vi "Main.vi"() -> ()   [LabVIEW 2022 SP3]
doc: "This template is for the Queued Message Handler design pattern.\n\nThe Event Handling Loop generates messages based on user interface actions.\n\nThe Message Handling Loop processes messages generated by the Event Handling Loop, or by other messages. The messages are string values, so new messages can be added easily to the Message Cases case structure in the Message Handling Loop. Each message cluster can also provide an optional value for Message Data, which is a variant that can be converted to whatever message-specific data is required."
uses:
  controls/UI Data.ctl
  support/Message Queue/Enqueue Message (Single).vi
  <vilib>/Utility/error.llb/Error Cluster From Error Code.vi
  <vilib>/ErrorRing/Error Ring.xnode
  support/Message Queue/Message Queue.lvlib
  support/User Event - Stop/User Event - Stop.lvlib
  support/User Event - ConnectionEvent/User Event - ConnectionEvent.lvlib
panel:
  out "sensors":dbl[](array[numeric])
  in  "Clear Console":bool
  in  "Restart Remote":bool
  in  "Network DAQ Rate (ms)":u32=500
  in  "Ignition Safety":bool
  in  "Ignition":bool
  in  "Deactuate 5":bool
  in  "Deactuate 4":bool
  in  "Deactuate 3":bool
  in  "Deactuate 2":bool
  in  "Deactuate 1":bool
  in  "Actuate 5":bool
  in  "Actuate 4":bool
  in  "Actuate 3":bool
  in  "Actuate 2":bool
  out "Ignition State":bool
  out "Switch 5":bool
  out "Switch 4":bool
  out "Switch 3":bool
  out "Switch 2":bool
  out "Switch 1":bool
  out "Pressure Transducers":waveform(dbl)[](graph)
  out "Temperature":waveform(dbl)[](graph)
  out "Load Cells & Strain Gauges":waveform(dbl)[](graph)
  out "Console":string
  in  "Disconnect":bool
  in  "Port":dbl=25005.0
  in  "IP Address":string="192.168.1.114"
  in  "Actuate 1":bool
  in  "Connect":bool
  in  "Exit":bool
  # "LC 0"
  # "LC 1"
  # "LC 2"
  # "LC 3"
  # "SG 0"
  # "SG 1"
  # "TC 0"
  # "TC 1"
  # "TC 2"
  # "TC 3"
  # "PT 0"
  # "PT 1"
  # "PT 2"
  # "PT 3"
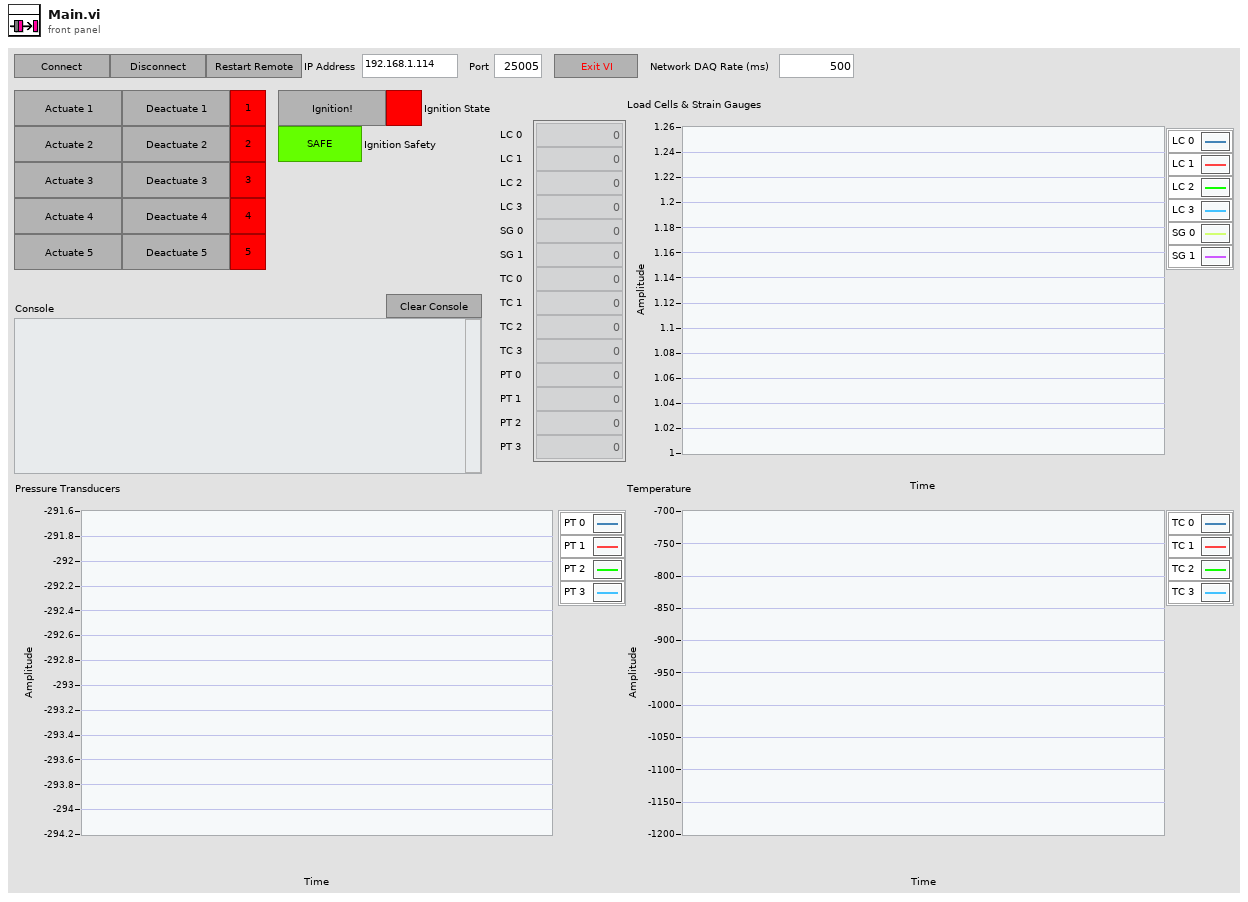
[diagram p1: front panel]
types:
  T1 = cluster{"ConnectionStatus":enum16{"Nothing", "Disconnect", "Connect", "Error"}}
  T2 = typedef "UI Data.ctl" = cluster{"Connect Ref":refnum<vi>, "Disconnect Ref":refnum<vi>, "Console Ref":refnum<vi>, "Exit Button Ref":refnum<vi>, "TCP Network Connection Refnum":refnum<k5>}
  T3 = typedef "Message Queue.lvlib/All Message Queues.ctl" = cluster{"UI":refnum<queue>}
  T4 = cluster{"command":string, "driver":i32, "value":i32}
  T5 = cluster{"[0]":bool, "[1]":bool, "[2]":bool, "[3]":bool, "[4]":bool, "[5]":bool, "[6]":bool, "[7]":bool, "[8]":bool}
  T6 = enum16{"Nothing", "Disconnect", "Connect", "Error"}
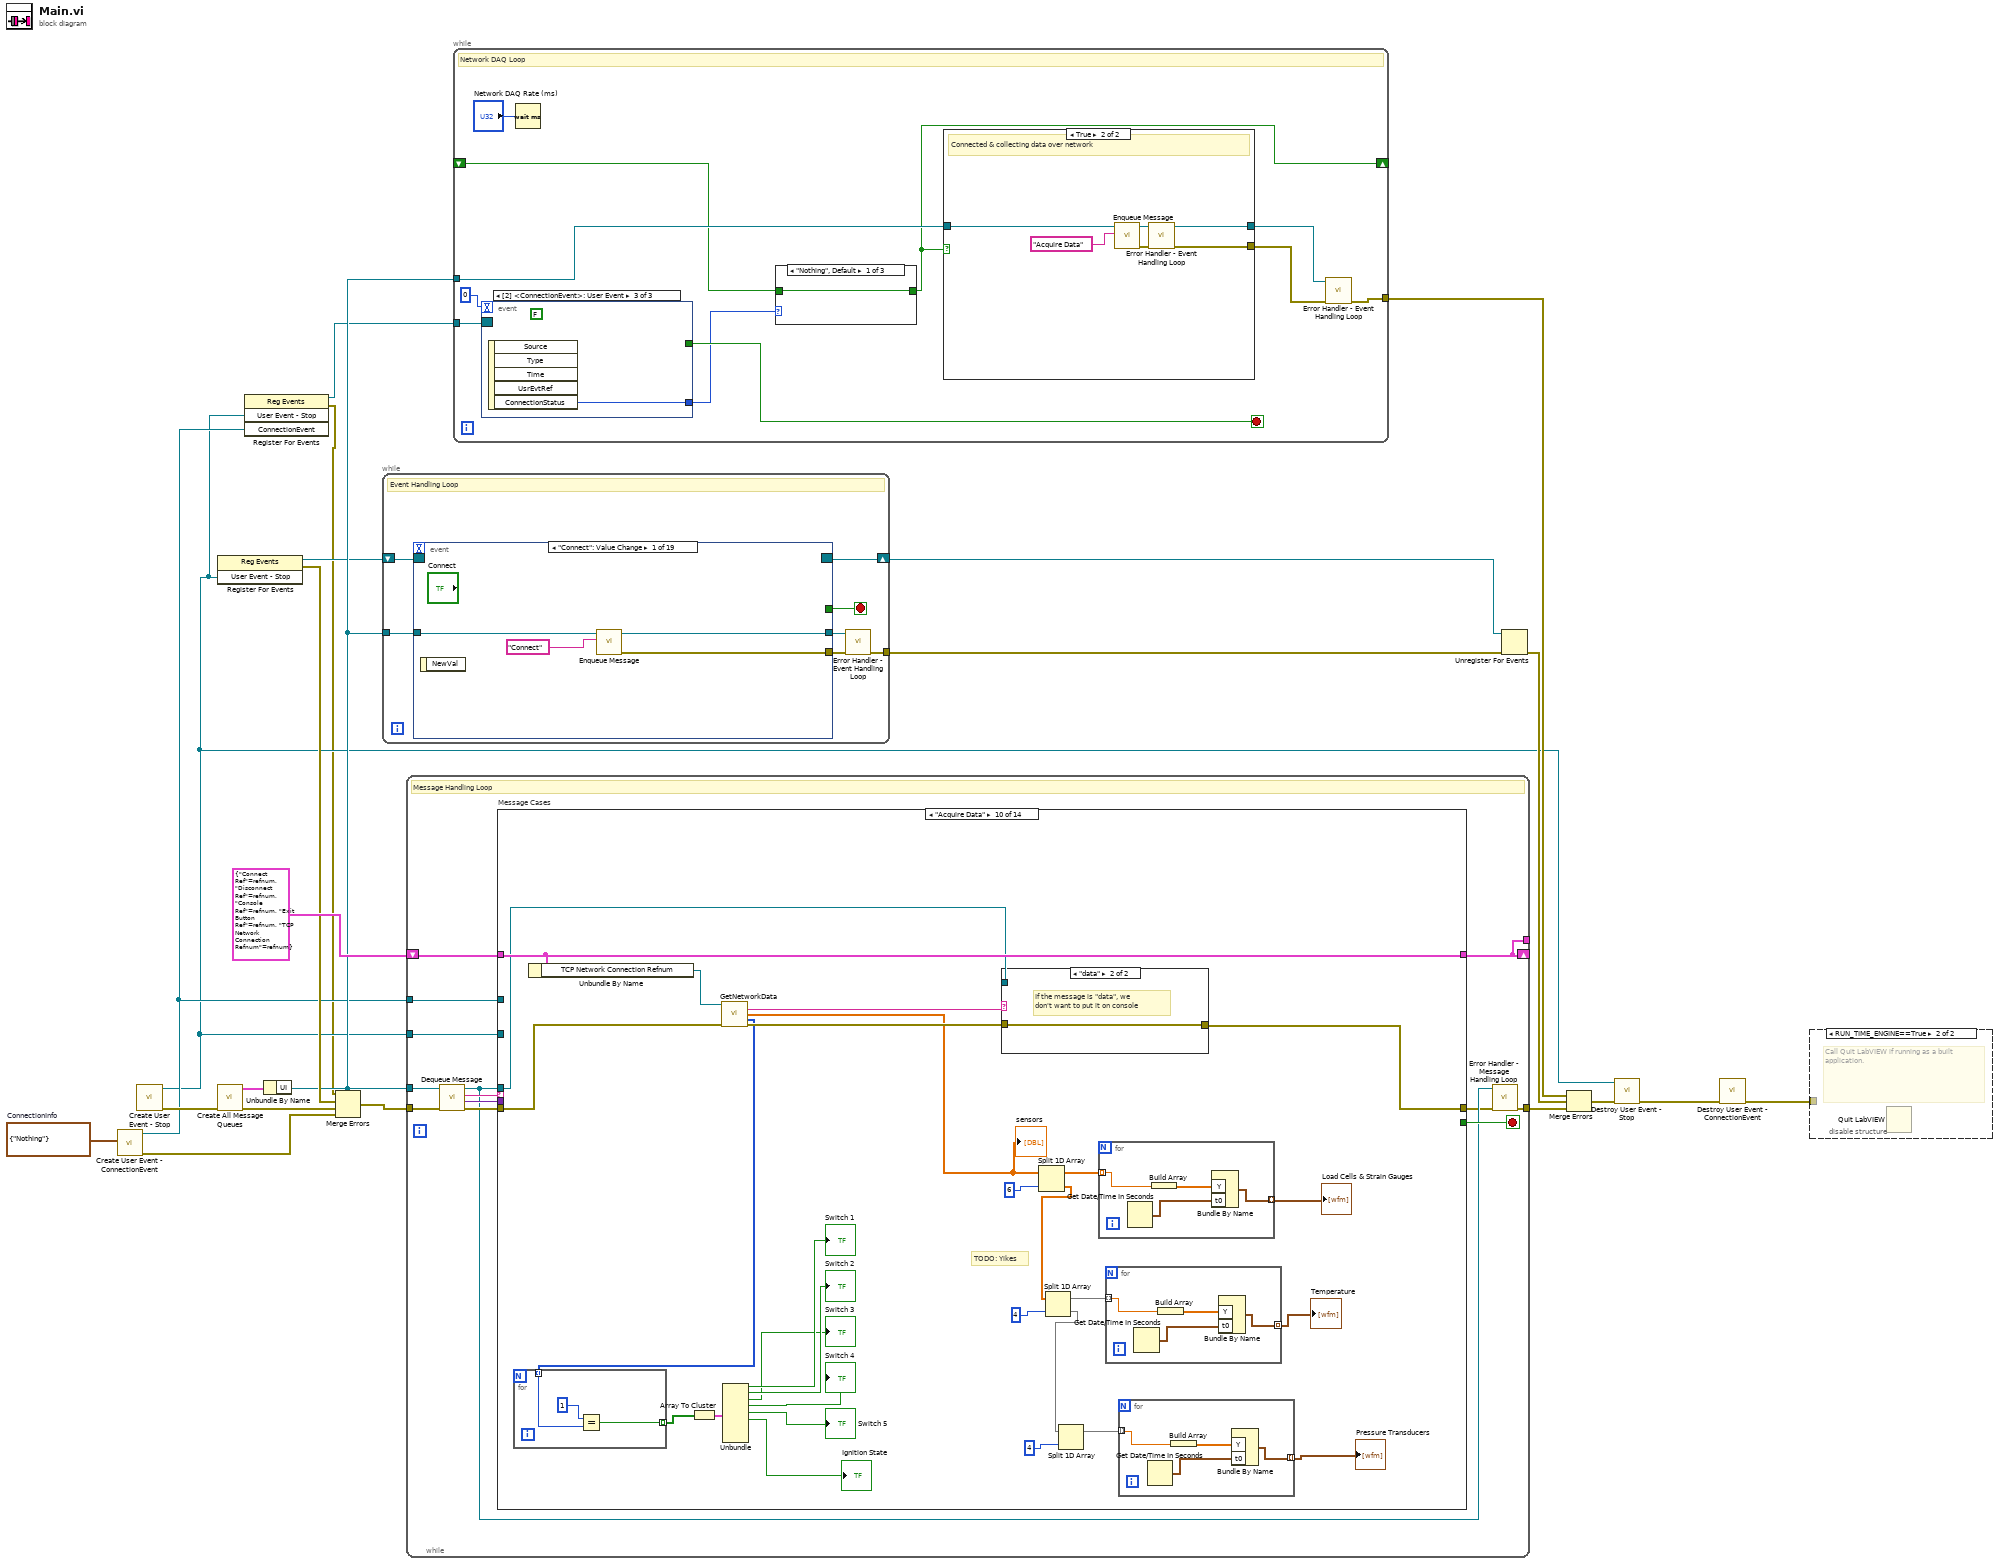
[diagram p0: block diagram]
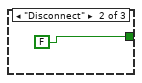
[diagram p2: hidden frame]
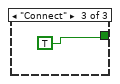
[diagram p3: hidden frame]
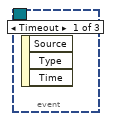
[diagram p4: hidden frame]
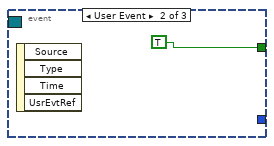
[diagram p5: hidden frame]
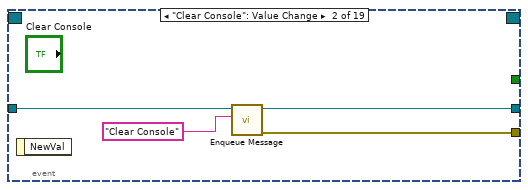
[diagram p8: hidden frame]
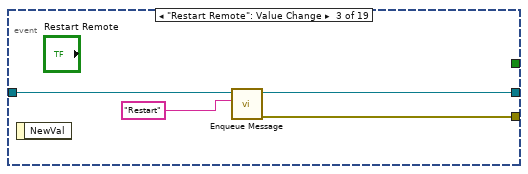
[diagram p9: hidden frame]
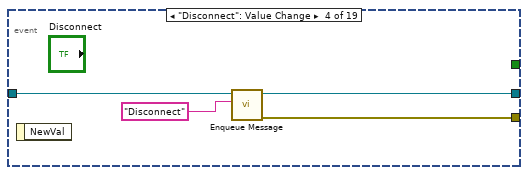
[diagram p10: hidden frame]
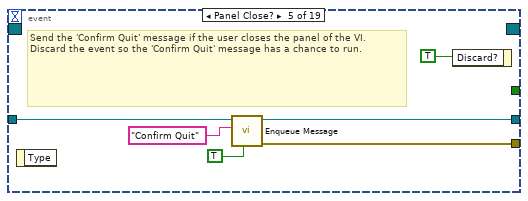
[diagram p11: hidden frame]
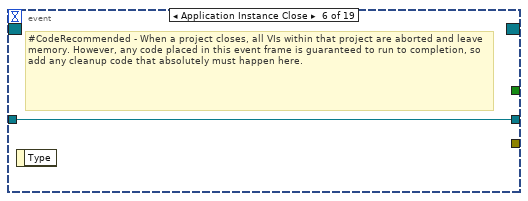
[diagram p12: hidden frame]
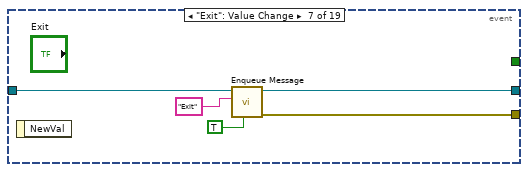
[diagram p13: hidden frame]
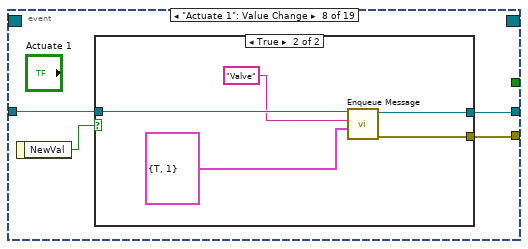
[diagram p14: hidden frame]
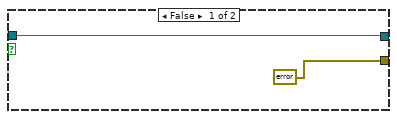
[diagram p15: hidden frame]
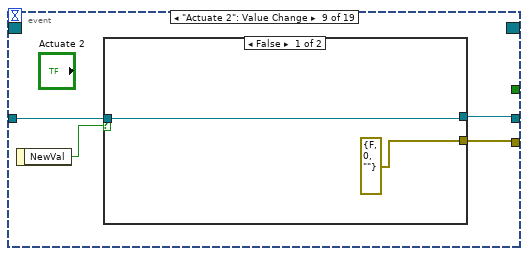
[diagram p16: hidden frame]
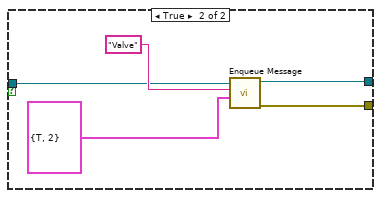
[diagram p17: hidden frame]
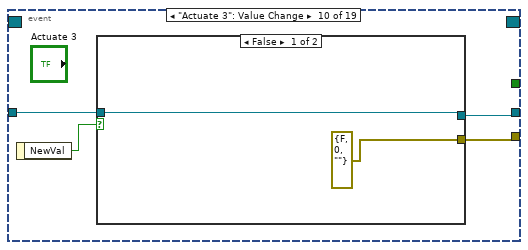
[diagram p18: hidden frame]
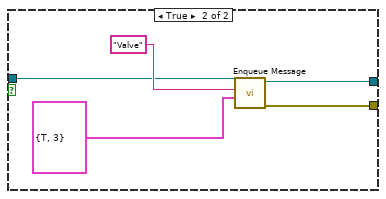
[diagram p19: hidden frame]
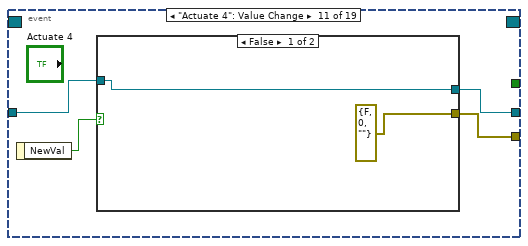
[diagram p20: hidden frame]
diagram:
  w5 = T1 {"ConnectionStatus"=enum."Nothing"}  # ConnectionInfo
  n1 = call "Create User Event - ConnectionEvent.vi"("ConnectionInfo"=w5) -> ("error out"=w6:errorcluster, "ConnectionEvent"=w4:refnum<user-event>)  [unwired: 9 in]
  n2 = call "Create User Event - Stop.vi"() -> ("error out"=w19:errorcluster, "User Event - Stop"=w3:refnum<user-event>)  [unwired: 10 in]
  n3 = call "Create All Message Queues.vi"("error in (no error)"=w19) -> ("error out"=w22:errorcluster, "Message Queues out"=w21:T3)  [unwired: 9 in]
  n4 = register-events(w3) -> (reference out=w9:refnum<event-registration>, error out=w12:errorcluster)  [unwired: 2 in]
  n5 = register-events(w3, w4) -> (reference out=w2:refnum<event-registration>, error out=w1:errorcluster)  [unwired: 2 in]
  n6 = Unbundle By Name(w21) -> ("UI"=w10:refnum<queue>)
  n7 = Merge Errors(w1, w12, w22, w6) -> (w13:errorcluster)
  n8 = while {
    tunnel: w10 -> [w29]
    shift-right: [w27] -> w16
    shift-left: w9 -> [w28]
    tunnel: [w23] -> w14
    stop <- w25 stop-if-true
    # "Event Handling Loop"
    n9 = event shown="[0] \"Connect\": Value Change" {
      selector: w28 -> [_ _ _ _ _ _ _ _ _ _ _ _ _ _ _ _ _ _ _]
      dyn-events: [_ _ _ _ _ _ _ _ _ _ _ _ _ _ _ _ _ _ _] -> w27
      timeout: _ -> [_ _ _ _ _ _ _ _ _ _ _ _ _ _ _ _ _ _ _]
      tunnel: [_ _ _ _ _ _ _ _ _ _ _ _ _ _ _ _ _ _ TRUE ("Discard?")] -> w25
      tunnel: w29 -> [w33 w37 w41 w45 w50 w52 w57 w61 w72 w83 w94 w105 w116 w127 w138 w149 w160 w171 w181]
      tunnel: [w30 w34 w38 w42 w49 _ w56 w59 w70 w81 w92 w103 w114 w125 w136 w147 w158 w169 _] -> w26
      tunnel: [w32 w36 w40 w44 w48 w52 w55 w60 w71 w82 w93 w104 w115 w126 w137 w148 w159 w170 w181] -> w24
      event "Connect": Value Change {
        n10 = event-data() -> ()  [unwired: 1 in, 1 out]
        n11 = call-poly "Enqueue Message.vi"("Message"="Connect", "Message Queue"=w33) -> ("error out"=w30:errorcluster, "dup Message Queue"=w32:refnum<queue>)  [unwired: 8 in]
      }
      event "Clear Console": Value Change {
        n12 = event-data() -> ()  [unwired: 1 in, 1 out]
        n13 = call-poly "Enqueue Message.vi"("Message"="Clear Console", "Message Queue"=w37) -> ("error out"=w34:errorcluster, "dup Message Queue"=w36:refnum<queue>)  [unwired: 8 in]
      }
      event "Restart Remote": Value Change {
        n14 = event-data() -> ()  [unwired: 1 in, 1 out]
        n15 = call-poly "Enqueue Message.vi"("Message"="Restart", "Message Queue"=w41) -> ("error out"=w38:errorcluster, "dup Message Queue"=w40:refnum<queue>)  [unwired: 8 in]
      }
      event "Disconnect": Value Change {
        n16 = event-data() -> ()  [unwired: 1 in, 1 out]
        n17 = call-poly "Enqueue Message.vi"("Message"="Disconnect", "Message Queue"=w45) -> ("error out"=w42:errorcluster, "dup Message Queue"=w44:refnum<queue>)  [unwired: 8 in]
      }
      event Panel Close? {
        # "Send the 'Confirm Quit' message if the user closes the panel of the VI. Discard the event so the 'Confirm Quit' message has a chance to run."
        n18 = event-data() -> ()  [unwired: 1 in, 1 out]
        n19 = call-poly "Enqueue Message.vi"("Priority Message? (F)"=TRUE, "Message"="Confirm Quit", "Message Queue"=w50) -> ("error out"=w49:errorcluster, "dup Message Queue"=w48:refnum<queue>)  [unwired: 7 in]
        n20 = event-data("Discard?"=TRUE) -> ()  [unwired: 1 in, 1 out]
      }
      event Application Instance Close {
        # "#CodeRecommended - When a project closes, all VIs within that project are aborted and leave memory. However, any code placed in this event frame is guaranteed to run to completion, so add any cleanup code that absolutely must happen here."
        n21 = event-data() -> ()  [unwired: 1 in, 1 out]
      }
      event "Exit": Value Change {
        n22 = event-data() -> ()  [unwired: 1 in, 1 out]
        n23 = call-poly "Enqueue Message.vi"("Priority Message? (F)"=TRUE, "Message"="Exit", "Message Queue"=w57) -> ("error out"=w56:errorcluster, "dup Message Queue"=w55:refnum<queue>)  [unwired: 7 in]
      }
      event "Actuate 1": Value Change {
        n24 = event-data() -> ("NewVal"=w58:bool)  [unwired: 1 in]
        n25 = case shown="True" w58 {
          tunnel: w61 -> [w63 w68]
          tunnel: [w63 w67] -> w60
          tunnel: [errorcluster {"status"=FALSE, "code"=0, "source"=""} ("error constant") w64] -> w59
          frame False {
          }
          frame True {
            n26 = call-poly "Enqueue Message.vi"("Message Data"=cluster{"Actuate?":bool, "Valve":i32} {"Actuate?"=TRUE, "Valve"=1}, "Message"="Valve", "Message Queue"=w68) -> ("error out"=w64:errorcluster, "dup Message Queue"=w67:refnum<queue>)  [unwired: 7 in]
          }
        }
      }
      event "Actuate 2": Value Change {
        n27 = event-data() -> ("NewVal"=w69:bool)  [unwired: 1 in]
        n28 = case shown="False" w69 {
          tunnel: w72 -> [w74 w77]
          tunnel: [w74 w76] -> w71
          tunnel: [errorcluster {"status"=FALSE, "code"=0, "source"=""} ("error constant") w75] -> w70
          frame False {
          }
          frame True {
            n29 = call-poly "Enqueue Message.vi"("Message Data"=cluster{"Actuate?":bool, "Valve":i32} {"Actuate?"=TRUE, "Valve"=2}, "Message"="Valve", "Message Queue"=w77) -> ("error out"=w75:errorcluster, "dup Message Queue"=w76:refnum<queue>)  [unwired: 7 in]
          }
        }
      }
      event "Actuate 3": Value Change {
        n30 = event-data() -> ("NewVal"=w80:bool)  [unwired: 1 in]
        n31 = case shown="False" w80 {
          tunnel: w83 -> [w85 w88]
          tunnel: [w85 w87] -> w82
          tunnel: [errorcluster {"status"=FALSE, "code"=0, "source"=""} ("error constant") w86] -> w81
          frame False {
          }
          frame True {
            n32 = call-poly "Enqueue Message.vi"("Message Data"=cluster{"Actuate?":bool, "Valve":i32} {"Actuate?"=TRUE, "Valve"=3}, "Message"="Valve", "Message Queue"=w88) -> ("error out"=w86:errorcluster, "dup Message Queue"=w87:refnum<queue>)  [unwired: 7 in]
          }
        }
      }
      event "Actuate 4": Value Change {
        n33 = event-data() -> ("NewVal"=w91:bool)  [unwired: 1 in]
        n34 = case shown="False" w91 {
          tunnel: w94 -> [w96 w99]
          tunnel: [w96 w98] -> w93
          tunnel: [errorcluster {"status"=FALSE, "code"=0, "source"=""} ("error constant") w97] -> w92
          frame False {
          }
          frame True {
            n35 = call-poly "Enqueue Message.vi"("Message Data"=cluster{"Actuate?":bool, "Valve":i32} {"Actuate?"=TRUE, "Valve"=4}, "Message"="Valve", "Message Queue"=w99) -> ("error out"=w97:errorcluster, "dup Message Queue"=w98:refnum<queue>)  [unwired: 7 in]
          }
        }
      }
      event "Actuate 5": Value Change {
        n36 = event-data() -> ("NewVal"=w102:bool)  [unwired: 1 in]
        n37 = case shown="False" w102 {
          tunnel: w105 -> [w107 w110]
          tunnel: [w107 w109] -> w104
          tunnel: [errorcluster {"status"=FALSE, "code"=0, "source"=""} ("error constant") w108] -> w103
          frame False {
          }
          frame True {
            n38 = call-poly "Enqueue Message.vi"("Message Data"=cluster{"Actuate?":bool, "Valve":i32} {"Actuate?"=TRUE, "Valve"=5}, "Message"="Valve", "Message Queue"=w110) -> ("error out"=w108:errorcluster, "dup Message Queue"=w109:refnum<queue>)  [unwired: 7 in]
          }
        }
      }
      event "Deactuate 1": Value Change {
        n39 = event-data() -> ("NewVal"=w113:bool)  [unwired: 1 in]
        n40 = case shown="False" w113 {
          tunnel: w116 -> [w118 w123]
          tunnel: [w118 w122] -> w115
          tunnel: [errorcluster {"status"=FALSE, "code"=0, "source"=""} ("error constant") w120] -> w114
          frame False {
          }
          frame True {
            n41 = call-poly "Enqueue Message.vi"("Message Data"=cluster{"Actuate?":bool, "Valve":i32} {"Actuate?"=FALSE, "Valve"=1}, "Message"="Valve", "Message Queue"=w123) -> ("error out"=w120:errorcluster, "dup Message Queue"=w122:refnum<queue>)  [unwired: 7 in]
          }
        }
      }
      event "Deactuate 2": Value Change {
        n42 = event-data() -> ("NewVal"=w124:bool)  [unwired: 1 in]
        n43 = case shown="False" w124 {
          tunnel: w127 -> [w129 w134]
          tunnel: [w129 w133] -> w126
          tunnel: [errorcluster {"status"=FALSE, "code"=0, "source"=""} ("error constant") w131] -> w125
          frame False {
          }
          frame True {
            n44 = call-poly "Enqueue Message.vi"("Message Data"=cluster{"Actuate?":bool, "Valve":i32} {"Actuate?"=FALSE, "Valve"=2}, "Message"="Valve", "Message Queue"=w134) -> ("error out"=w131:errorcluster, "dup Message Queue"=w133:refnum<queue>)  [unwired: 7 in]
          }
        }
      }
      event "Deactuate 3": Value Change {
        n45 = event-data() -> ("NewVal"=w135:bool)  [unwired: 1 in]
        n46 = case shown="False" w135 {
          tunnel: w138 -> [w140 w145]
          tunnel: [w140 w144] -> w137
          tunnel: [errorcluster {"status"=FALSE, "code"=0, "source"=""} ("error constant") w142] -> w136
          frame False {
          }
          frame True {
            n47 = call-poly "Enqueue Message.vi"("Message Data"=cluster{"Actuate?":bool, "Valve":i32} {"Actuate?"=FALSE, "Valve"=3}, "Message"="Valve", "Message Queue"=w145) -> ("error out"=w142:errorcluster, "dup Message Queue"=w144:refnum<queue>)  [unwired: 7 in]
          }
        }
      }
      event "Deactuate 4": Value Change {
        n48 = event-data() -> ("NewVal"=w146:bool)  [unwired: 1 in]
        n49 = case shown="False" w146 {
          tunnel: w149 -> [w151 w156]
          tunnel: [w151 w155] -> w148
          tunnel: [errorcluster {"status"=FALSE, "code"=0, "source"=""} ("error constant") w153] -> w147
          frame False {
          }
          frame True {
            n50 = call-poly "Enqueue Message.vi"("Message Data"=cluster{"Actuate?":bool, "Valve":i32} {"Actuate?"=FALSE, "Valve"=4}, "Message"="Valve", "Message Queue"=w156) -> ("error out"=w153:errorcluster, "dup Message Queue"=w155:refnum<queue>)  [unwired: 7 in]
          }
        }
      }
      event "Deactuate 5": Value Change {
        n51 = event-data() -> ("NewVal"=w157:bool)  [unwired: 1 in]
        n52 = case shown="False" w157 {
          tunnel: w160 -> [w162 w167]
          tunnel: [w162 w166] -> w159
          tunnel: [errorcluster {"status"=FALSE, "code"=0, "source"=""} ("error constant") w164] -> w158
          frame False {
          }
          frame True {
            n53 = call-poly "Enqueue Message.vi"("Message Data"=cluster{"Actuate?":bool, "Valve":i32} {"Actuate?"=FALSE, "Valve"=5}, "Message"="Valve", "Message Queue"=w167) -> ("error out"=w164:errorcluster, "dup Message Queue"=w166:refnum<queue>)  [unwired: 7 in]
          }
        }
      }
      event "Ignition": Value Change {
        n54 = event-data() -> ()  [unwired: 1 in, 1 out]
        n55 = case shown="False" "Ignition Safety" {
          tunnel: w171 -> [w174 w179]
          tunnel: [w174 w178] -> w170
          tunnel: [errorcluster {"status"=FALSE, "code"=0, "source"=""} ("error constant") w176] -> w169
          frame False {
            n56 = One Button Dialog(message="UNSAFE before attempting ignition.") -> ()  [unwired: 1 in, 1 out]
          }
          frame True {
            n57 = call-poly "Enqueue Message.vi"("Message Data"=cluster{"Actuate?":bool, "Valve":i32} {"Actuate?"=TRUE, "Valve"=6}, "Message"="Valve", "Message Queue"=w179) -> ("error out"=w176:errorcluster, "dup Message Queue"=w178:refnum<queue>)  [unwired: 7 in]
          }
        }
      }
      event User Event {
        # "The Message Handling Loop processed an \"Exit\" message, which fired this event to stop the Event Handling Loop."
        n58 = event-data() -> ()  [unwired: 1 in, 1 out]
      }
    }
    n59 = call "Error Handler - Event Handling Loop.vi"("error in (no error)"=w26, "Message Queue"=w24) -> ("dup error in"=w23:errorcluster)  [unwired: 8 in, 1 out]
  }
  n60 = while {
    tunnel: w10 -> [w188]
    shift-right: [w184] -> _
    shift-left: T2 {"Connect Ref"=refnum, "Disconnect Ref"=refnum, "Console Ref"=refnum, "Exit Button Ref"=refnum, "TCP Network Connection Refnum"=refnum} ("Data Cluster") -> [w182]
    tunnel: w3 -> [w193]
    tunnel: w13 -> [w192]
    tunnel: [w186] -> w20
    tunnel: [w184] -> _
    tunnel: w4 -> [w183]
    stop <- w194 stop-if-true
    # "Message Handling Loop"
    n61 = call "Dequeue Message.vi"("error in (no error)"=w192, "Message Queue"=w188) -> ("error out"=w191:errorcluster, "Message Data"=w189:variant, "Message"=w190:string, "dup Message Queue"=w187:refnum<queue>)  [unwired: 6 in]
    n62 = case "Message Cases" shown="\"Acquire Data\"" w190 {
      selector: w190 -> [_ _ _ _ _ _ _ _ _ _ _ _ _ w379]
      tunnel: w187 -> [w199 w205 w233 w246 _ _ w273 _ _ w309 w354 w359 w378 _]
      tunnel: w191 -> [w203 w224 w241 w248 w261 w270 w277 w280 w284 w285 w346 w366 w371 _]
      tunnel: [w204 w211 w238 w249 w262 w264 w275 w278 w282 w286 w356 w360 w374 w380] -> w185
      tunnel: w182 -> [w202 w217 w235 w250 w263 w269 w276 w279 w283 w312 w352 w363 w377 w381]
      tunnel: [w201 w216 w235 w250 w263 w269 w276 w279 w283 w312 w352 w363 w377 w381] -> w184
      tunnel: [_ _ _ _ _ _ _ _ _ _ _ _ TRUE _] -> w194
      tunnel: w189 -> [_ _ _ _ w260 w268 _ _ _ _ w347 _ w368 _]
      tunnel: w193 -> [_ _ _ _ _ _ _ _ _ _ _ _ w373 _]
      tunnel: w183 -> [_ w209 w242 _ _ _ _ _ _ _ _ _ _ _]
      frame "Initialize" {
        # "Initialize - All initialization work should take place in this message, since other loops can potentially enqueue messages that execute immediately after this one."
        n63 = control-ref of="Connect"() -> (w197:refnum<vi>)
        n64 = control-ref of="Exit"() -> (w196:refnum<vi>)
        n65 = control-ref of="Console"() -> (w195:refnum<vi>)
        n66 = Bundle By Name(cluster=w202, "Connect Ref"=w197, "Console Ref"=w195, "Exit Button Ref"=w196) -> (w201:T2)
        n67 = call-poly "Enqueue Message.vi"("error in (no error)"=w203, "Message Data"="Initial Message" ("Initial Message"), "Message"="Update Console", "Message Queue"=w199) -> ("error out"=w204:errorcluster)  [unwired: 6 in, 1 out]
      }
      frame "Connect" {
        w210 = T1 {"ConnectionStatus"=enum."Connect"}  # ConnectionInfo
        # "Connect to the specified port & IP and send timestamp over network.\nTODO: Disable IP & port controls when connected, possibly grey out everything\nelse when not connected\nTODO: Properly handle error when connecting"
        # "Something - Replace this message with functionality for your own application."
        n68 = TCP Open Connection(address="IP Address", remote port or service name="Port", error in (no error)=w224) -> (connection ID=w218:refnum<k5>, error out=w207:errorcluster)  [unwired: 2 in]
        n69 = case shown="Error .." w207 {
          tunnel: [_ w232] -> w206
          tunnel: w205 -> [_ w229]
          frame No Error {
          }
          frame Error {
            n70 = call-poly "Enqueue Message.vi"("Message Data"="Failed to connect to remote" ("\"Do Something\" button pressed"), "Message"="Update Console", "Message Queue"=w229) -> ("error out"=w230:errorcluster, "dup Message Queue"=w228:refnum<queue>)  [unwired: 7 in]
            n71 = call-poly "Enqueue Message.vi"("Priority Message? (F)"=TRUE, "error in (no error)"=w230, "Message"="Exit", "Message Queue"=w228) -> ("error out"=w232:errorcluster)  [unwired: 6 in, 1 out]
          }
        }
        n72 = Get Date/Time In Seconds() -> (seconds since 1Jan1904=w223:timestamp)
        n73 = To Double Precision Float(number=w223) -> (double precision float=w222:dbl)
        n74 = Number To Decimal String(number=w222) -> (decimal integer string=w221:string)  [unwired: 1 in]
        n75 = TCP Write(connection ID=w218, data in=w221, error in (no error)=w206) -> (connection ID out=w215:refnum<k5>, error out=w208:errorcluster)  [unwired: 1 in, 1 out]
        n76 = Bundle By Name(cluster=w217, "TCP Network Connection Refnum"=w215) -> (w216:T2)
        n77 = call "Fire User Event - ConnectionEvent.vi"("error in (no error)"=w208, "ConnectionInfo"=w210, "ConnectionEvent"=w209) -> ("error out"=w212:errorcluster)  [unwired: 8 in]
        n78 = call-poly "Enqueue Message.vi"("error in (no error)"=w212, "Message Data"="Connected to remote." ("\"Do Something\" button pressed"), "Message"="Update Console", "Message Queue"=w205) -> ("error out"=w211:errorcluster)  [unwired: 6 in, 1 out]
      }
      frame "Disconnect" {
        w243 = T1 {"ConnectionStatus"=enum."Disconnect"}  # ConnectionInfo
        n79 = Unbundle By Name(w235) -> ("TCP Network Connection Refnum"=w234:refnum<k5>)
        n80 = call "Fire User Event - ConnectionEvent.vi"("error in (no error)"=w241, "ConnectionInfo"=w243, "ConnectionEvent"=w242) -> ("error out"=w237:errorcluster)  [unwired: 8 in]
        n81 = TCP Close Connection(connection ID=w234, error in (no error)=w237) -> (error out=w236:errorcluster)  [unwired: 1 in, 1 out]
        n82 = call-poly "Enqueue Message.vi"("error in (no error)"=w236, "Message Data"="Disconnected from remote." ("\"Do Something\" button pressed"), "Message"="Update Console", "Message Queue"=w233) -> ("error out"=w238:errorcluster)  [unwired: 6 in, 1 out]
      }
      frame "Something Else" {
        # "Send string to \"Update Display\" message"
        # "#CodeNeeded - Perform whatever actions correspond to the \"Something Else\" message."
        # "Something Else - Replace this message with functionality for your own application."
        n83 = call-poly "Enqueue Message.vi"("error in (no error)"=w248, "Message Data"="\"Do Something Else\" button pressed" ("\"Do Something Else\" button pressed"), "Message"="Update Display", "Message Queue"=w246) -> ("error out"=w247:errorcluster)  [unwired: 6 in, 1 out]
        n84 = Merge Errors(w247) -> (w249:errorcluster)
      }
      frame "Update Console" {
        # "Append new line to current console output"
        # "Update Display - Convert the message data to a string to display in the Data Display indicator."
        n85 = Variant To Data(error in=w261, type="", Variant=w260) -> (data=w256:string, error out=w258:errorcluster)
        n86 = property on="Console" class="Str"() -> ("Text.Text"=w253:string)  [unwired: 2 in, 2 out]
        n87 = Concatenate Strings(w253, "\r\n", w256) -> (→"Console":string)
        n88 = Merge Errors(w258) -> (w262:errorcluster)
        n89 = call <vilib>:"Delimited String to 1D String Array.vi"("delimiter"="\r\n", "delimited string"=w253) -> ("string array"=w252:string[])  [unwired: 9 in]
        n90 = Array Size(array=w252) -> (size(s)=w251:i32)
        n91 = property on="Console" class="Str"("Text.Scroll Position"=w251) -> ()  [unwired: 2 in, 2 out]
      }
      frame "Error" {
        # "#CodeRecommended - If you ever change the name of this \"Error\" message, you'll need to update the name in the Check Loop Error.vi as well."
        # "#CodeRecommended - Consider creating a system for logging errors in some way. These errors are for notification purposes only. Handling of specific errors should be performed in the message frames that generated the error."
        # "Error - Display an error dialog. This message is sent by the \"Error Handler\" VIs at the end of other loops in this application."
        n92 = Variant To Data(error in=w270, type=errorcluster {"status"=FALSE, "code"=0, "source"=""} ("error constant"), Variant=w268) -> (data=w266:errorcluster, error out=w265:errorcluster)
        n93 = call <vilib>:"Simple Error Handler.vi"("error in (no error)"=w266) -> ()  [unwired: 4 in, 5 out]
        n94 = Merge Errors(w265) -> (w264:errorcluster)
      }
      frame "Confirm Quit" {
        # "#CodeNeeded - If you want to provide an \"Are you sure\" dialog (or some other notification) before the application exits, place that code here. This message is typically sent from a Panel Close? event."
        # "Confirm Quit - Message that can confirm whether or not the user wants to exit the application."
        n95 = call-poly "Enqueue Message.vi"("Priority Message? (F)"=TRUE, "error in (no error)"=w277, "Message"="Exit", "Message Queue"=w273) -> ("error out"=w274:errorcluster)  [unwired: 6 in, 1 out]
        n96 = Merge Errors(w274) -> (w275:errorcluster)
      }
      frame "---Copy This Frame---" {
        # "Duplicate this frame when creating new messages.  Change this comment in the duplicated frame to describe this message."
        n97 = Merge Errors(w280) -> (w278:errorcluster)
      }
      frame "Clear Console" {
        # "Duplicate this frame when creating new messages.  Change this comment in the duplicated frame to describe this message."
        n98 = property on="Console" class="Str"("Text.Text"="") -> ()  [unwired: 2 in, 2 out]
        n99 = Merge Errors(w284) -> (w282:errorcluster)
      }
      frame "Acquire Data" {
        # "TODO: Yikes"
        # "Duplicate this frame when creating new messages.  Change this comment in the duplicated frame to describe this message."
        n100 = Unbundle By Name(w312) -> ("TCP Network Connection Refnum"=w311:refnum<k5>)
        n101 = call "GetNetworkData.vi"("TCP Network Connection in"=w311, "error in (no error)"=w285) -> ("console"=w310:string, "sensors"=w296:dbl[], "states"=w287:i32[], "error out"=w308:errorcluster)  [unwired: 9 in, 1 out]
        "sensors" <- w296
        n102 = for {
          tunnel: w287 -> [w314] mode=indexing
          tunnel: [w313] -> w289 mode=indexing
          n103 = Equal?(x=1, y=w314) -> (x = y?=w313:bool)
        }
        n104 = Array To Cluster(array=w289) -> (cluster=w288:T5)
        n105 = Unbundle(w288) -> ("[0]"=→"Switch 1":bool, "[1]"=→"Switch 2":bool, "[2]"=→"Switch 3":bool, "[3]"=→"Switch 4":bool, "[4]"=→"Switch 5":bool, "[5]"=→"Ignition State":bool)  [unwired: 3 out]
        n106 = case shown="\"data\"" w310 {
          selector: w310 -> [w329 _]
          tunnel: w309 -> [w332 _]
          tunnel: w308 -> [w331 w333]
          tunnel: [w330 w333] -> w286
          frame Default {
            n107 = call-poly "Enqueue Message.vi"("error in (no error)"=w331, "Message Data"=w329, "Message"="Update Console", "Message Queue"=w332) -> ("error out"=w330:errorcluster)  [unwired: 6 in, 1 out]
          }
          frame "data" {
            # "If the message is \"data\", we\ndon't want to put it on console"
          }
        }
        n108 = Split 1D Array(array=w296, index=6) -> (first subarray=w306:dbl[], second subarray=w302:dbl[])
        n109 = Split 1D Array(array=w302, index=4) -> (first subarray=w303:dbl[], second subarray=w298:dbl[])
        n110 = Split 1D Array(array=w298, index=4) -> (first subarray=w299:dbl[])  [unwired: 1 out]
        n111 = for {
          tunnel: w306 -> [w326] mode=indexing
          tunnel: [w324] -> w305 mode=indexing
          n112 = Get Date/Time In Seconds() -> (seconds since 1Jan1904=w327:timestamp)
          n113 = Build Array(w326) -> (w325:dbl[])
          n114 = Bundle By Name("Y"=w325, "t0"=w327) -> (w324:waveform(dbl))  [unwired: 1 in]
        }
        "Load Cells & Strain Gauges" <- w305
        n115 = for {
          tunnel: w303 -> [w322] mode=indexing
          tunnel: [w320] -> w301 mode=indexing
          n116 = Get Date/Time In Seconds() -> (seconds since 1Jan1904=w323:timestamp)
          n117 = Build Array(w322) -> (w321:dbl[])
          n118 = Bundle By Name("Y"=w321, "t0"=w323) -> (w320:waveform(dbl))  [unwired: 1 in]
        }
        "Temperature" <- w301
        n119 = for {
          tunnel: w299 -> [w318] mode=indexing
          tunnel: [w316] -> w297 mode=indexing
          n120 = Get Date/Time In Seconds() -> (seconds since 1Jan1904=w319:timestamp)
          n121 = Build Array(w318) -> (w317:dbl[])
          n122 = Bundle By Name("Y"=w317, "t0"=w319) -> (w316:waveform(dbl))  [unwired: 1 in]
        }
        "Pressure Transducers" <- w297
      }
      frame "Valve" {
        # "Duplicate this frame when creating new messages.  Change this comment in the duplicated frame to describe this message."
        n123 = Variant To Data(error in=w346, type=cluster{"Actuate?":bool, "Valve":i32} {"Actuate?"=TRUE, "Valve"=1}, Variant=w347) -> (data=w344:cluster{"Actuate?":bool, "Valve":i32})  [unwired: 1 out]
        n124 = Unbundle By Name(w344) -> ("Valve"=w340:i32, "Actuate?"=w343:bool)
        n125 = Unbundle By Name(w352) -> ("TCP Network Connection Refnum"=w349:refnum<k5>)
        n126 = Boolean To (0,1)(Boolean=w343) -> (0, 1=w337:i16)
        n127 = Bundle By Name(cluster=T4 {"command"="set_valve", "driver"=0, "value"=1}, "driver"=w340, "value"=w337) -> (w348:T4)
        n128 = Flatten To JSON(anything=w348) -> (JSON string=w334:string, 11:w351:errorcluster)  [unwired: 2 in]
        n129 = TCP Write(connection ID=w349, data in=w334, error in (no error)=w351) -> (error out=w350:errorcluster)  [unwired: 1 in, 2 out]
        n130 = Number To Decimal String(number=w337) -> (decimal integer string=w338:string)  [unwired: 1 in]
        n131 = Number To Decimal String(number=w340) -> (decimal integer string=w341:string)  [unwired: 1 in]
        n132 = Concatenate Strings("COMMAND: set_valve (driver = " ("\"Do Something\" button pressed"), w341, ", value = ", w338, ")") -> (w336:string)
        n133 = call-poly "Enqueue Message.vi"("error in (no error)"=w350, "Message Data"=w336, "Message"="Update Console", "Message Queue"=w354) -> ("error out"=w356:errorcluster)  [unwired: 6 in, 1 out]
      }
      frame "Restart" {
        n134 = Unbundle By Name(w363) -> ("TCP Network Connection Refnum"=w362:refnum<k5>)
        n135 = Flatten To JSON(anything=cluster{"command":string} {"command"="close"}, error in (no error)=w366) -> (JSON string=w364:string, 11:w367:errorcluster)  [unwired: 1 in]
        n136 = TCP Write(connection ID=w362, data in=w364, error in (no error)=w367) -> (error out=w361:errorcluster)  [unwired: 1 in, 2 out]
        n137 = call-poly "Enqueue Message.vi"("error in (no error)"=w361, "Message Data"="COMMAND: shutdown", "Message"="Update Console", "Message Queue"=w359) -> ("error out"=w360:errorcluster)  [unwired: 6 in, 1 out]
      }
      frame "Exit" {
        # "TODO: Clear console? Maybe j add clear console button?"
        # "Stop the VI"
        # "Release the message queue reference"
        # "#CodeNeeded - Add any required cleanup code here. Note that if 'Exit' was called as a result of an error, an error dialog will be displayed. Add any custom error handling for an 'Exit' condition here as well."
        # "Exit - Exit the application."
        n138 = Variant To Data(type=errorcluster {"status"=FALSE, "code"=0, "source"=""} ("error constant"), Variant=w368) -> (data=w369:errorcluster)  [unwired: 1 in, 1 out]
        n139 = call <vilib>:"Simple Error Handler.vi"("error in (no error)"=w369) -> ()  [unwired: 4 in, 5 out]
        n140 = call "Fire User Event - Stop.vi"("User Event - Stop"=w373) -> ("error out"=w372:errorcluster)  [unwired: 10 in]
        n141 = Release Queue(queue=w378, error in (no error)=w371) -> (error out=w375:errorcluster)  [unwired: 1 in, 2 out]
        n142 = Merge Errors(w372, w375) -> (w374:errorcluster)
      }
      frame Default {
        # "'Default' case only runs if there is a message that isn't defined in any of the other cases.  Output a programming error."
        n143 = xnode "Error Ring"("parameter 0"=w379) -> ("error out"=w380:errorcluster)
      }
    }
    n144 = call "Error Handler - Message Handling Loop.vi"("error in (no error)"=w185, "Message Queue"=w187) -> ("dup error in"=w186:errorcluster)  [unwired: 8 in, 1 out]
  }
  n145 = while {
    tunnel: w10 -> [w399]
    tunnel: [w391] -> w11
    tunnel: w2 -> [w395]
    shift-right: [w392] -> _
    shift-left: _ -> [w393]
    stop <- w396 stop-if-true
    (unwired) FALSE
    # "Network DAQ Loop"
    n146 = event shown="[2] <ConnectionEvent>: User Event" {
      selector: w395 -> [_ _ _]
      dyn-events: _ -> [_ _ _]
      timeout: 0 -> [_ _ _]
      tunnel: [_ TRUE _] -> w396
      tunnel: [_ _ w404] -> w394
      event Timeout {
        n147 = event-data() -> ()  [unwired: 1 in, 3 out]
      }
      event User Event {
        n148 = event-data() -> ()  [unwired: 1 in, 4 out]
      }
      event User Event {
        n149 = event-data() -> ("ConnectionStatus"=w404:T6)  [unwired: 1 in, 4 out]
      }
    }
    n150 = Wait (ms)(milliseconds to wait="Network DAQ Rate (ms)") -> ()  [unwired: 1 out]
    n151 = case shown="\"Nothing\", Default" w394 {
      tunnel: [w400 FALSE TRUE] -> w392
      tunnel: w393 -> [w400 _ _]
      frame "Nothing", Default {
      }
      frame "Disconnect" {
      }
      frame "Connect" {
      }
    }
    n152 = case shown="True" w392 {
      tunnel: w399 -> [w405 w410]
      tunnel: [_ w407] -> w390
      tunnel: [w405 w406] -> w389
      frame False {
      }
      frame True {
        # "Connected & collecting data over network"
        n153 = call-poly "Enqueue Message.vi"("Message"="Acquire Data", "Message Queue"=w410) -> ("error out"=w408:errorcluster, "dup Message Queue"=w409:refnum<queue>)  [unwired: 8 in]
        n154 = call "Error Handler - Event Handling Loop.vi"("error in (no error)"=w408, "Message Queue"=w409) -> ("dup error in"=w407:errorcluster, "dup Message Queue"=w406:refnum<queue>)  [unwired: 8 in]
      }
    }
    n155 = call "Error Handler - Event Handling Loop.vi"("error in (no error)"=w390, "Message Queue"=w389) -> ("dup error in"=w391:errorcluster)  [unwired: 8 in, 1 out]
  }
  n156 = Unregister For Events(event registration refnum=w16, error in=w14) -> (error out=w17:errorcluster)
  n157 = Merge Errors(w11, w17, w20) -> (w18:errorcluster)
  n158 = call "Destroy User Event - Stop.vi"("error in (no error)"=w18, "User Event - Stop"=w3) -> ("error out"=w7:errorcluster)  [unwired: 9 in]
  n159 = call "Destroy User Event - ConnectionEvent.vi"("error in (no error)"=w7) -> ("error out"=w8:errorcluster)  [unwired: 10 in]
  n160 = disable-structure shown="RUN_TIME_ENGINE==True" {
    disable-tunnel: w8 -> [_ _]
    frame condition #0 (active) {
    }
    frame condition #1 {
      # "Call Quit LabVIEW if running as a built application."
      n161 = Quit LabVIEW() -> ()  [unwired: 1 in]
    }
  }
